vi "Stop&Close.vi"(8 "error in (no error)":errorcluster) -> (0 "error out":errorcluster)   [LabVIEW 2014, in "OPCUA Server(UtilityMode)(dev).lvlib"]
uses:
  OPCUA Server(UtilityMode)(dev).lvlib
  _op(server).ctl
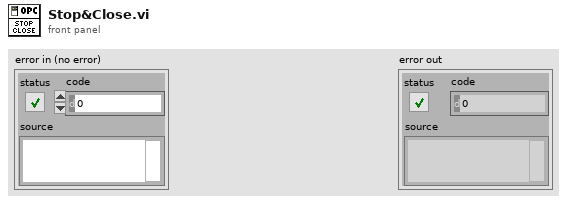
[diagram p1: front panel]
types:
  T1 = typedef "OPCUA Server(UtilityMode)(dev).lvlib/_op(server).ctl" = enum16{"Create Server", "Start Server", "Get Server Refnum", "Stop Server", "Close Server"}
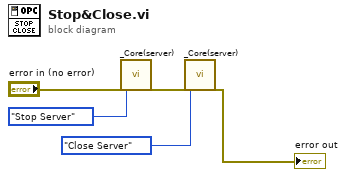
[diagram p0: block diagram]
diagram:
  n1 = call "_Core(server).vi"("error in (no error)"="error in (no error)", "Op"=_op(server)."Stop Server") -> ("error out"=w2:errorcluster)  [unwired: 21 in, 4 out]
  n2 = call "_Core(server).vi"("error in (no error)"=w2, "Op"=_op(server)."Close Server") -> ("error out"=→"error out":errorcluster)  [unwired: 21 in, 4 out]
